vi "DataLog File Metrics.vi"(7 "point index":dbl) -> (3 "index in chunk":i32, 4 "points left in chunk":i32, 6 "chunk index":i32, 8 "log file index":i32, 10 "log file offset":i32, 15 "at chunk boundary?":bool)   [LabVIEW 2012]
doc: "Calculate some chunk/file metrics given a point index."
uses:
  glb_DataLog MCVD.vi
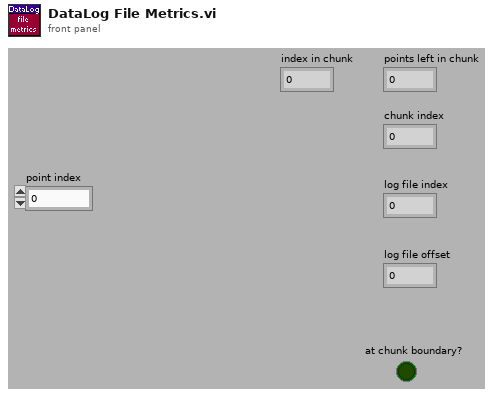
[diagram p1: front panel]
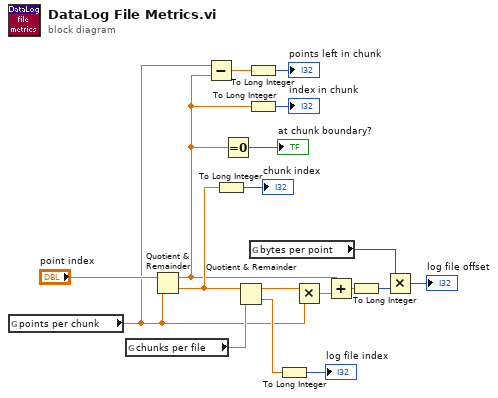
[diagram p0: block diagram]
diagram:
  n1 = global read "glb_DataLog MCVD.vi" "points per chunk"() -> (w9:dbl)
  n2 = global read "glb_DataLog MCVD.vi" "chunks per file"() -> (w18:dbl)
  n3 = Quotient & Remainder(x="point index", y=w9) -> (x-y*floor(x/y)=w2:dbl, floor(x/y)=w14:dbl)
  n4 = Subtract(x=w9, y=w2) -> (x-y=w16:dbl)
  n5 = To Long Integer(number=w14) -> (32bit integer=→"chunk index":i32)
  n6 = Equal To 0?(x=w2) -> (x = 0?=→"at chunk boundary?":bool)
  n7 = Quotient & Remainder(x=w14, y=w18) -> (x-y*floor(x/y)=w10:dbl, floor(x/y)=w11:dbl)
  n8 = To Long Integer(number=w16) -> (32bit integer=→"points left in chunk":i32)
  n9 = To Long Integer(number=w2) -> (32bit integer=→"index in chunk":i32)
  n10 = global read "glb_DataLog MCVD.vi" "bytes per point"() -> (w1:i32)
  n11 = To Long Integer(number=w11) -> (32bit integer=→"log file index":i32)
  n12 = Multiply(x=w10, y=w9) -> (x*y=w8:dbl)
  n13 = Add(x=w2, y=w8) -> (x+y=w7:dbl)
  n14 = To Long Integer(number=w7) -> (32bit integer=w6:i32)
  n15 = Multiply(x=w1, y=w6) -> (x*y=→"log file offset":i32)
